vi "Laser Constraints.vi"(6 "Dac Min":u16, 7 "DAC Max":u16, 8 "error in (no error)":errorcluster, 9 "Thold Low":u16, 10 "Thold HI":u16, 11 "Select Probe":i32) -> (0 "error out":errorcluster)   [LabVIEW 2015, in "Tool Interface.lvlib"]
uses:
  Tool Interface.lvlib
  Tool Typedefs/_Laser Constraints Cluster--typedef.ctl
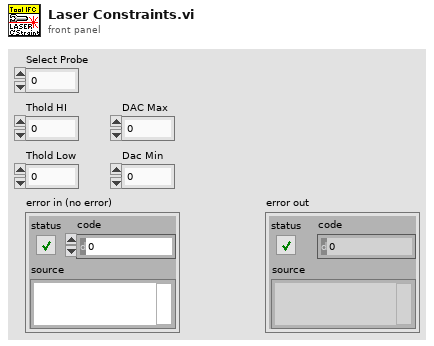
[diagram p1: front panel]
types:
  T1 = typedef "_Laser Constraints Cluster--typedef.ctl" = cluster{"Mode":i16, "Thold Low":u16, "Thold High":u16, "DAC Min":u16, "DAC Max":u16}
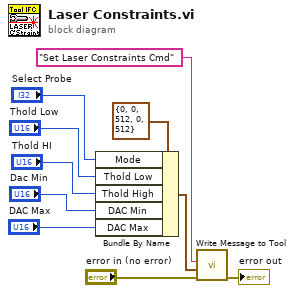
[diagram p0: block diagram]
diagram:
  n1 = Bundle By Name(cluster=T1 {"Mode"=0, "Thold Low"=0, "Thold High"=512, "DAC Min"=0, "DAC Max"=512} ("_Laser Constraints Cluster--typedef"), "Mode"="Select Probe", "Thold Low"="Thold Low", "Thold High"="Thold HI", "DAC Min"="Dac Min", "DAC Max"="DAC Max") -> (w6:T1)
  n2 = call "Write Message to Tool.vi"("error in (no error)"="error in (no error)", "Message Data"=w6, "Message"="Set Laser Constraints Cmd") -> ("error out"=→"error out":errorcluster)  [unwired: 8 in]
